vi "averageNframes.vi"(9 "first frame index":dbl, 10 "number of frames":dbl, 11 "Images In":T1[](array[typedef])) -> (3 "Image out":T1(plugin-control))   [LabVIEW 2009]
uses:
  <vilib>/vision/Image Controls.llb/IMAQ Image.ctl
panel:
  in  "Numeric 2":dbl
  in  "Numeric":dbl
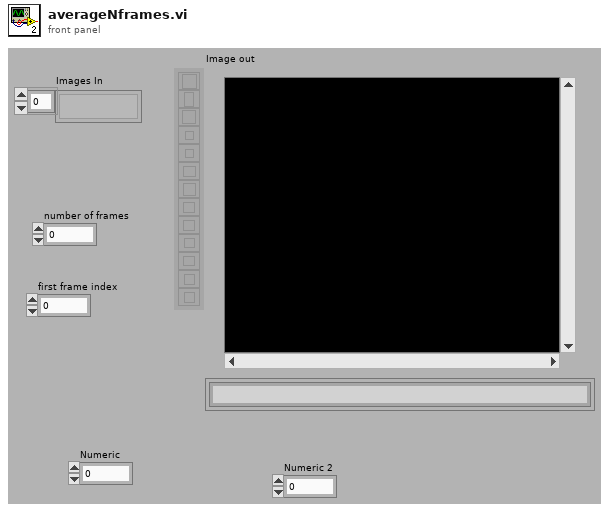
[diagram p1: front panel]
types:
  T1 = typedef "IMAQ Image.ctl" = refnum<image>
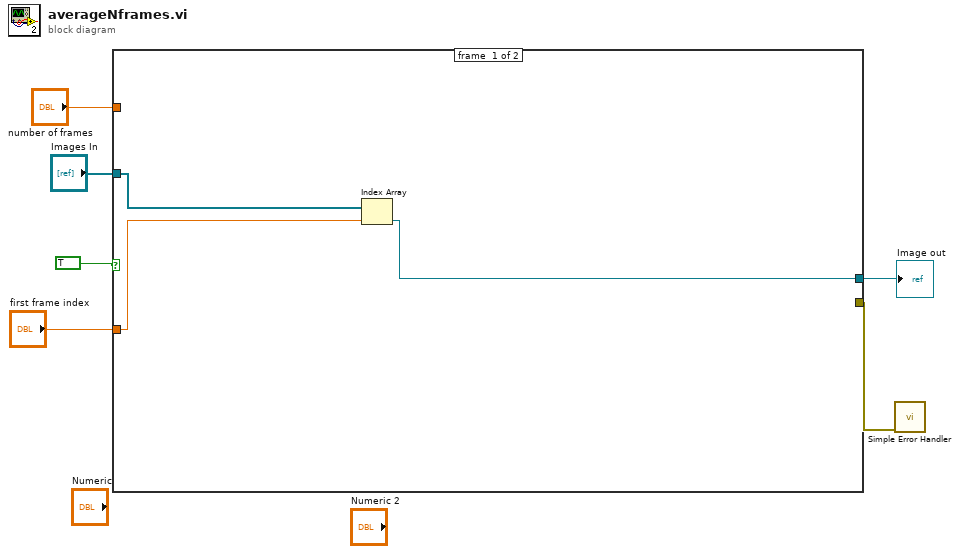
[diagram p0: block diagram]
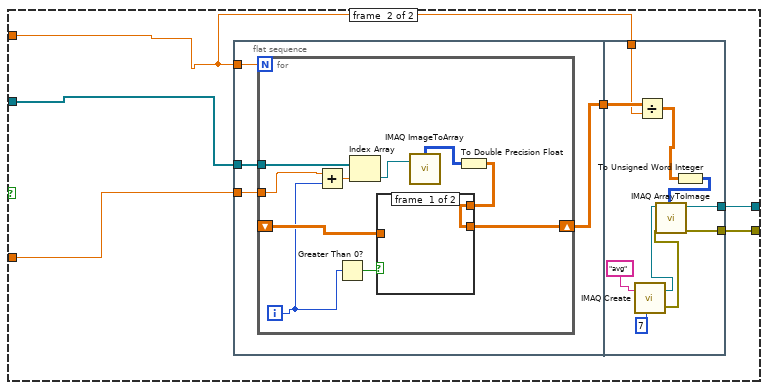
[diagram p2: hidden frame]
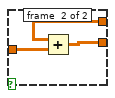
[diagram p3: hidden frame]
diagram:
  n1 = case shown="True" TRUE {
    tunnel: [w7 w14] -> w2
    tunnel: "Images In" -> [w8 w13]
    tunnel: "number of frames" -> [_ w12]
    tunnel: "first frame index" -> [w9 w11]
    tunnel: [_ w10] -> w1
    frame #0 {
      n2 = Index Array(array=w8, index=w9) -> (element=w7:T1)
    }
    frame #1 {
      n3 = flat-sequence {
        tunnel: w12 -> [w19]
        tunnel: w13 -> [w18]
        tunnel: w11 -> [w17]
        tunnel: [w16] -> w15
        tunnel: w15 -> [w43]
        tunnel: [w42] -> w14
        tunnel: w12 -> [w41]
        tunnel: [w39] -> w10
        frame #0 {
          n4 = for {
            N: w19 -> [_]
            tunnel: w18 -> [w21]
            tunnel: w17 -> [w28]
            shift-right: [w26] -> w16
            shift-left: _ -> [w25]
            i -> [w20]
            n5 = Add(x=w28, y=w20) -> (x+y=w29:dbl)
            n6 = Greater Than 0?(x=w20) -> (x > 0?=w24:bool)
            n7 = Index Array(array=w21, index=w29) -> (element=w22:T1)
            n8 = call "IMAQ ImageToArray"("Image"=w22) -> ("Image Pixels (U8)"=w23:u8[][])  [unwired: 3 in, 4 out]
            n9 = To Double Precision Float(number=w23) -> (double precision float=w27:dbl[][])
            n10 = case shown="True" w24 {
              tunnel: w27 -> [w30 w33]
              tunnel: [w30 w32] -> w26
              tunnel: w25 -> [_ w31]
              frame #0 {
              }
              frame #1 {
                n11 = Add(x=w33, y=w31) -> (x+y=w32:dbl[][])
              }
            }
          }
        }
        frame #1 {
          n12 = call "IMAQ Create"("Image Name"="avg", "Image Type"=7) -> ("New Image"=w35:T1, "error out"=w34:errorcluster)  [unwired: 3 in]
          n13 = Divide(x=w43, y=w41) -> (x/y=w40:dbl[][])
          n14 = To Unsigned Word Integer(number=w40) -> (unsigned 16bit integer=w38:u16[][])
          n15 = call "IMAQ ArrayToImage"("Image Pixels (U16)"=w38, "error in (no error)"=w34, "Image"=w35) -> ("error out"=w39:errorcluster, "Image Out"=w42:T1)  [unwired: 7 in]
        }
      }
    }
  }
  "Image out" <- w2
  n16 = call <vilib>:"Simple Error Handler.vi"("error in (no error)"=w1) -> ()  [unwired: 4 in, 5 out]
